vi "Create Basic Response.vi"(8 "error in (no error)":errorcluster, 9 "Content-Type (text/plain)":string="text/plain", 10 "Payload":string, 11 "Status Code":u16) -> (0 "error out":errorcluster, 3 "Response out":refnum<class "Response.lvclass">)   [LabVIEW 2020, in "HTTP Utils.lvlib" / "Response.lvclass"]
uses:
  Response.lvclass
  Response.lvclass/Response.ctl
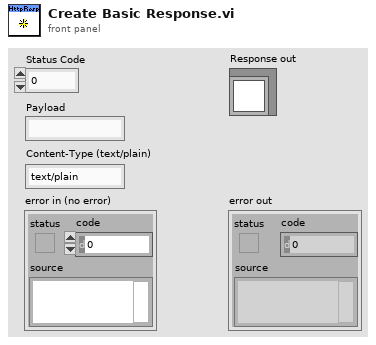
[diagram p1: front panel]
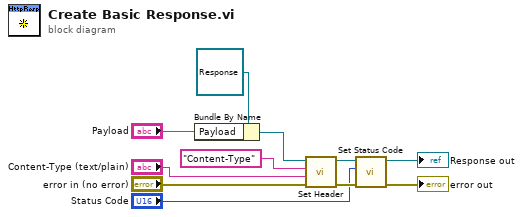
[diagram p0: block diagram]
diagram:
  n1 = Bundle By Name(cluster=refnum<class "Response.lvclass"> refnum ("Response in"), "Payload"="Payload") -> (w8:refnum<class "Response.lvclass">)
  n2 = call "Set Header.vi"("error in (no error)"="error in (no error)", "Value"="Content-Type (text/plain)", "Header"="Content-Type", "Response in"=w8) -> ("error out"=w4:errorcluster, "Response out"=w5:refnum<class "Response.lvclass">)  [unwired: 5 in, 1 out]
  n3 = call "Set Status Code.vi"("error in (no error)"=w4, "Status Code"="Status Code", "Response in"=w5) -> ("error out"=→"error out":errorcluster, "Response out"=→"Response out":refnum<class "Response.lvclass">)  [unwired: 7 in]
